vi "DetermineRegimeTest.vi"() -> (3 "Were there any errors at all?":bool)   [LabVIEW 2013]
uses:
  Data/TypeDefs/Sailing Regimes.ctl
  Data/TypeDefs/Boat Regimes.ctl
  Data/TypeDefs/Emergency Regimes.ctl
panel:
  in  "Input regimes (Last commanded)":T1[](array[typedef])=[{"Sailing Regime"=enum."Tack - Bow across wind", "Emergency Regimes"=enum."NO EMERGENCY", "Emergency?"=FALSE}, {"Sailing Regime"=enum."Upwind - Starboard Tack", "Emergency Regimes"=enum."NO EMERGENCY", "Emergency?"=FALSE}, {"Sailing Regime"=enum."Upwind - Port Tack", "Emergency Regimes"=enum."NO EMERGENCY", "Emergency?"=FALSE}, {"Sailing Regime"=enum."Jibe - Stern across wind", "Emergency Regimes"=enum."NO EMERGENCY", "Emergency?"=FALSE}, {"Sailing Regime"=enum."Upwind - Starboard Tack", "Emergency Regimes"=enum."NO EMERGENCY", "Emergency?"=FALSE}]
  out "Output regimes":T1[](array[typedef])=[{"Sailing Regime"=enum."Upwind - Starboard Tack", "Emergency Regimes"=enum."NO EMERGENCY", "Emergency?"=FALSE}, {"Sailing Regime"=enum."Turn between Upwind/Reach - Starboard Tack", "Emergency Regimes"=enum."NO EMERGENCY", "Emergency?"=FALSE}, {"Sailing Regime"=enum."Turn between Upwind/Reach - Port Tack", "Emergency Regimes"=enum."NO EMERGENCY", "Emergency?"=FALSE}, {"Sailing Regime"=enum."Jibe - Stern across wind", "Emergency Regimes"=enum."NO EMERGENCY", "Emergency?"=FALSE}, {"Sailing Regime"=enum."Upwind - Starboard Tack", "Emergency Regimes"=enum."NO EMERGENCY", "Emergency?"=FALSE}]
  in  "Desired Heading Input":dbl[](array[numeric])=[50.0, 65.0, 170.0, 10.0, 74.0, 0.0]
  in  "Expected regime outputs":T2[](array[typedef])=[enum."Upwind - Starboard Tack", enum."Turn between Upwind/Reach - Starboard Tack", enum."Turn between Upwind/Reach - Port Tack", enum."Jibe - Stern across wind", enum."Upwind - Starboard Tack", enum."Reach - Port Tack"]
  in  "Actual Heading Input":dbl[](array[numeric])=[50.0, 50.0, 310.0, 354.0, 69.0, 0.0]
  out "Are chosen regimes right?":bool[](array[boolean])=[TRUE, TRUE, TRUE, TRUE, TRUE]
  in  "Wind Inputs":dbl[](array[numeric])=[0.0, 0.0, 0.0, 180.0, 0.0, 76.0]
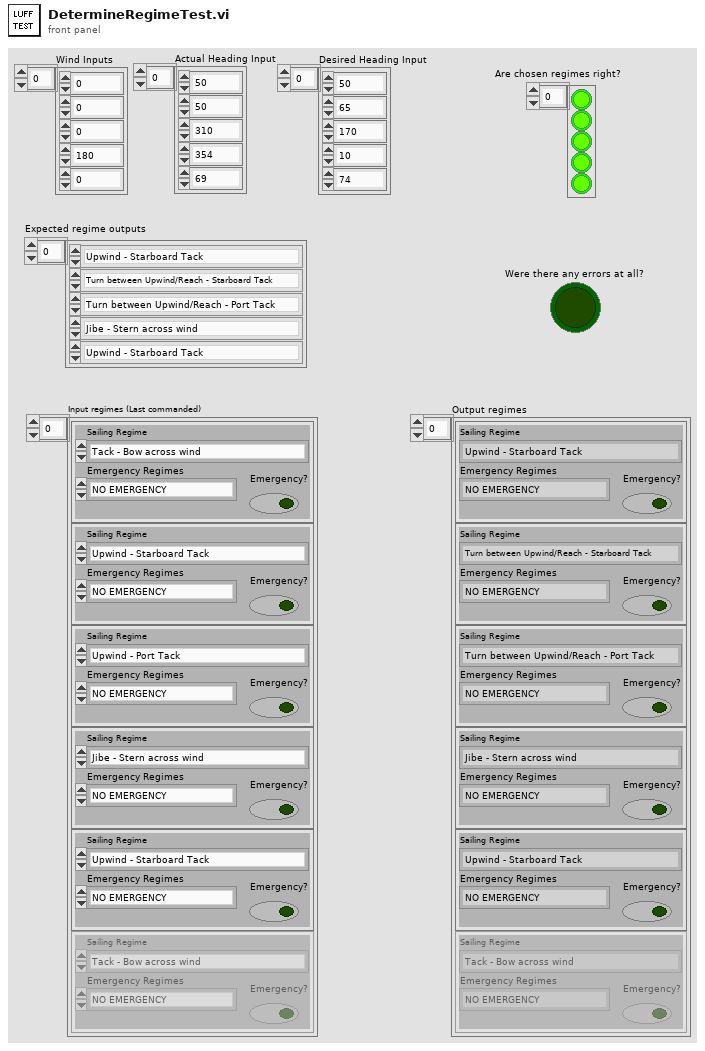
[diagram p1: front panel]
types:
  T1 = typedef "Boat Regimes.ctl" = cluster{"Sailing Regime":T2, "Emergency Regimes":T3, "Emergency?":bool}
  T2 = typedef "Sailing Regimes.ctl" = enum16{"Tack - Bow across wind", "Upwind - Starboard Tack", "Turn between Upwind/Reach - Starboard Tack", "Reach - Starboard Tack", "Turn between Reach/Run - Starboard Tack", "Run - Starboard Tack", "Jibe - Stern across wind", "Run - Port Tack", "Turn between Reach/Run - Port Tack", "Reach - Port Tack", "Turn between Upwind/Reach - Port Tack", "Upwind - Port Tack"}
  T3 = typedef "Emergency Regimes.ctl" = enum16{"NO EMERGENCY", "No Knockdown", "Obstacle Avoid"}
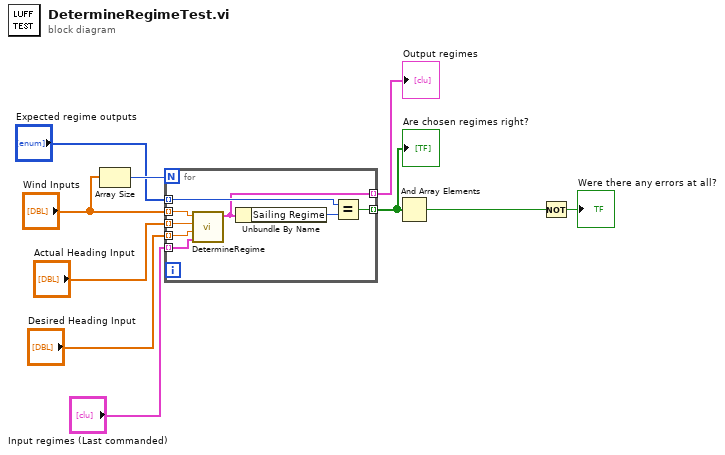
[diagram p0: block diagram]
diagram:
  n1 = Array Size(array="Wind Inputs") -> (size(s)=w10:i32)
  n2 = for {
    N: w10 -> [_]
    tunnel: "Wind Inputs" -> [w15] mode=indexing
    tunnel: "Expected regime outputs" -> [w18] mode=indexing
    tunnel: [w17] -> w8 mode=indexing
    tunnel: "Actual Heading Input" -> [w16] mode=indexing
    tunnel: "Desired Heading Input" -> [w14] mode=indexing
    tunnel: [w12] -> w2 mode=indexing
    tunnel: "Input regimes (Last commanded)" -> [w13] mode=indexing
    n3 = call "DetermineRegime.vi"("Last Commanded Boat Regime"=w13, "Desired Heading (deg)"=w14, "Robot Heading (deg)"=w16, "Trusted Absolute Wind Data (deg)"=w15) -> ("Commanded Boat Regime"=w12:T1)  [unwired: 7 in]
    n4 = Unbundle By Name(w12) -> ("Sailing Regime"=w11:T2)
    n5 = Equal?(x=w18, y=w11) -> (x = y?=w17:bool)
  }
  "Are chosen regimes right?" <- w8
  "Output regimes" <- w2
  n6 = And Array Elements(Boolean array=w8) -> (logical AND=w5:bool)
  n7 = Not(x=w5) -> (.not. x?=→"Were there any errors at all?":bool)
